vi "数据库读取子vi.vi"() -> (3 "Data":string[][](array[string]))   [LabVIEW 2014]
panel:
  out "error out":errorcluster
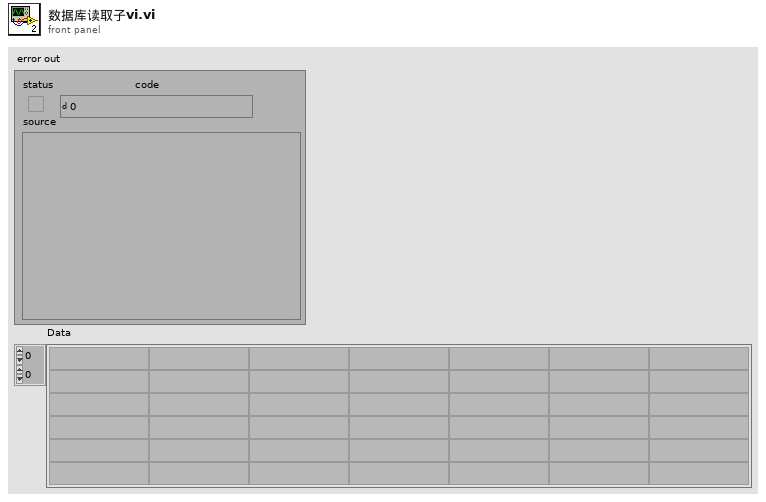
[diagram p1: front panel]
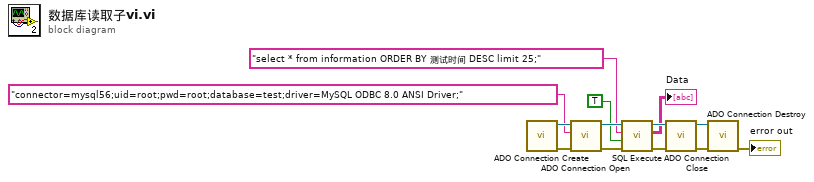
[diagram p0: block diagram]
diagram:
  n1 = call "ADO Connection Create.vi"() -> ("error out"=w12:errorcluster, "ADODB._Connection Out"=w13:refnum<k7>)  [unwired: 10 in]
  n2 = call "ADO Connection Open.vi"("error in (no error)"=w12, "ConnectionString"="connector=mysql56;uid=root;pwd=root;database=test;driver=MySQL ODBC 8.0 ANSI Driver;", "ADODB._Connection In"=w13) -> ("error out"=w10:errorcluster, "ADODB._Connection Out"=w11:refnum<k7>)  [unwired: 7 in]
  n3 = call "SQL Execute.vi"("error in (no error)"=w10, "Return Data (T)"=TRUE, "Command Text"="select * from information ORDER BY 测试时间 DESC limit 25;", "ADODB._Connection In"=w11) -> ("error out"=w8:errorcluster, "Data"=→"Data":string[][], "ADODB._Connection Out"=w9:refnum<k7>)  [unwired: 4 in, 1 out]
  n4 = call "ADO Connection Close.vi"("error in (no error)"=w8, "ADODB._Connection In"=w9) -> ("error out"=w6:errorcluster, "ADODB._Connection Out"=w7:refnum<k7>)  [unwired: 8 in]
  n5 = call "ADO Connection Destroy.vi"("error in (no error)"=w6, "ADODB._Connection In"=w7) -> ("error out"=→"error out":errorcluster)  [unwired: 9 in]
